vi "parse_TransformStamped_roslv.vi"(0 "msg in":string, 3 "error in":errorcluster) -> (5 "Transform":T1, 6 "msg out":string, 7 "Header":T2, 8 "child_frame_id":string, 9 "error out":errorcluster)   [LabVIEW 2014]
doc: "Parses a message into a transform stamped"
uses:
  std_msgs/subs/parse_string_scalar_roslv.vi
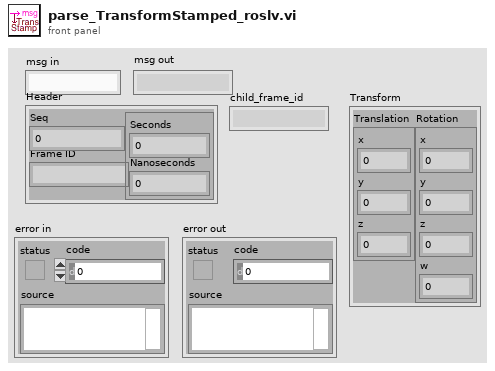
[diagram p1: front panel]
types:
  T1 = cluster{"Translation":cluster{"x":dbl, "y":dbl, "z":dbl}, "Rotation":cluster{"x":dbl, "y":dbl, "z":dbl, "w":dbl}}
  T2 = cluster{"Seq":u32, "Frame ID":string, "Timestamp":cluster{"Seconds":i32, "Nanoseconds":i32}}
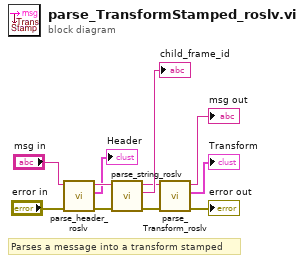
[diagram p0: block diagram]
diagram:
  # "Parses a message into a transform stamped"
  n1 = call "parse_header_roslv.vi"("error in"="error in", "msg in"="msg in") -> ("error out"=w8:errorcluster, "Header"=→"Header":T2, "msg out"=w9:string)  [unwired: 3 in]
  n2 = call-poly "parse_string_roslv.vi"("error in"=w8, "msg in"=w9) -> ("error out"=w4:errorcluster, "string"=→"child_frame_id":string, "msg out"=w5:string)  [unwired: 3 in]
  n3 = call "parse_Transform_roslv.vi"("error in"=w4, "msg in"=w5) -> ("error out"=→"error out":errorcluster, "Transform"=→"Transform":T1, "msg out"=→"msg out":string)  [unwired: 3 in]
